vi "Create_Graph_v1.4.vi"() -> ()   [LabVIEW 2018]
uses:
  <vilib>/Native 3D Graph/xcontrol/3DPC_SurfacePlot.xctl
  <vilib>/Native 3D Graph/classes/Base Datatype.lvclass
panel:
  out "3D Graph":refnum<class "Base Datatype.lvclass">[](xcontrol)
  out "Array 2":dbl[][](array[numeric])
  in  "Open":bool
  in  "Загрузка Excel приложения":refnum<k7>
  in  "Excel._Worksheet 2":refnum<k7>
  in  "Array":string[][](array[string])
  in  "Выбор файла":path
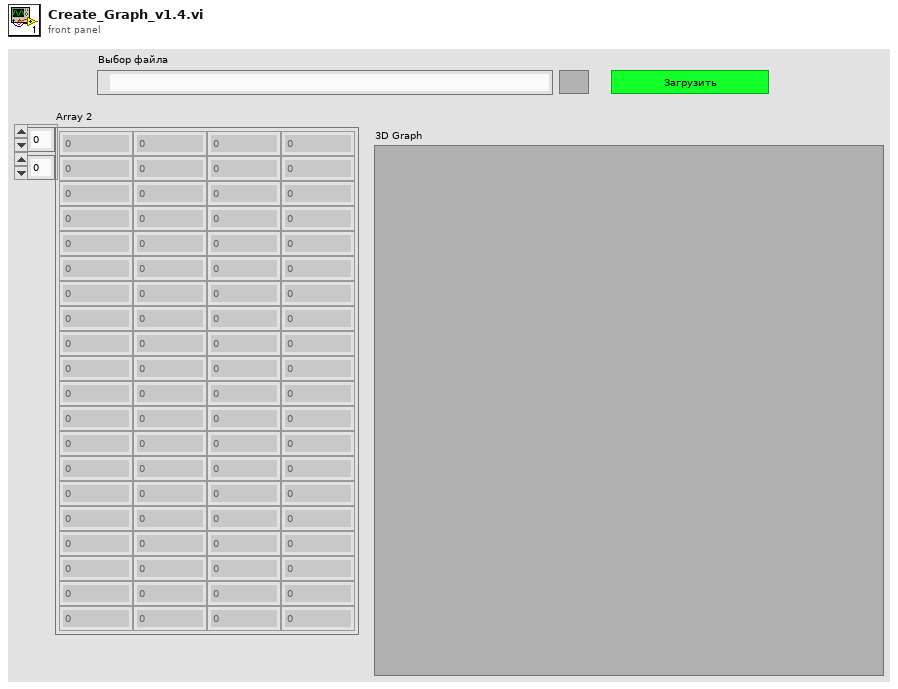
[diagram p1: front panel]
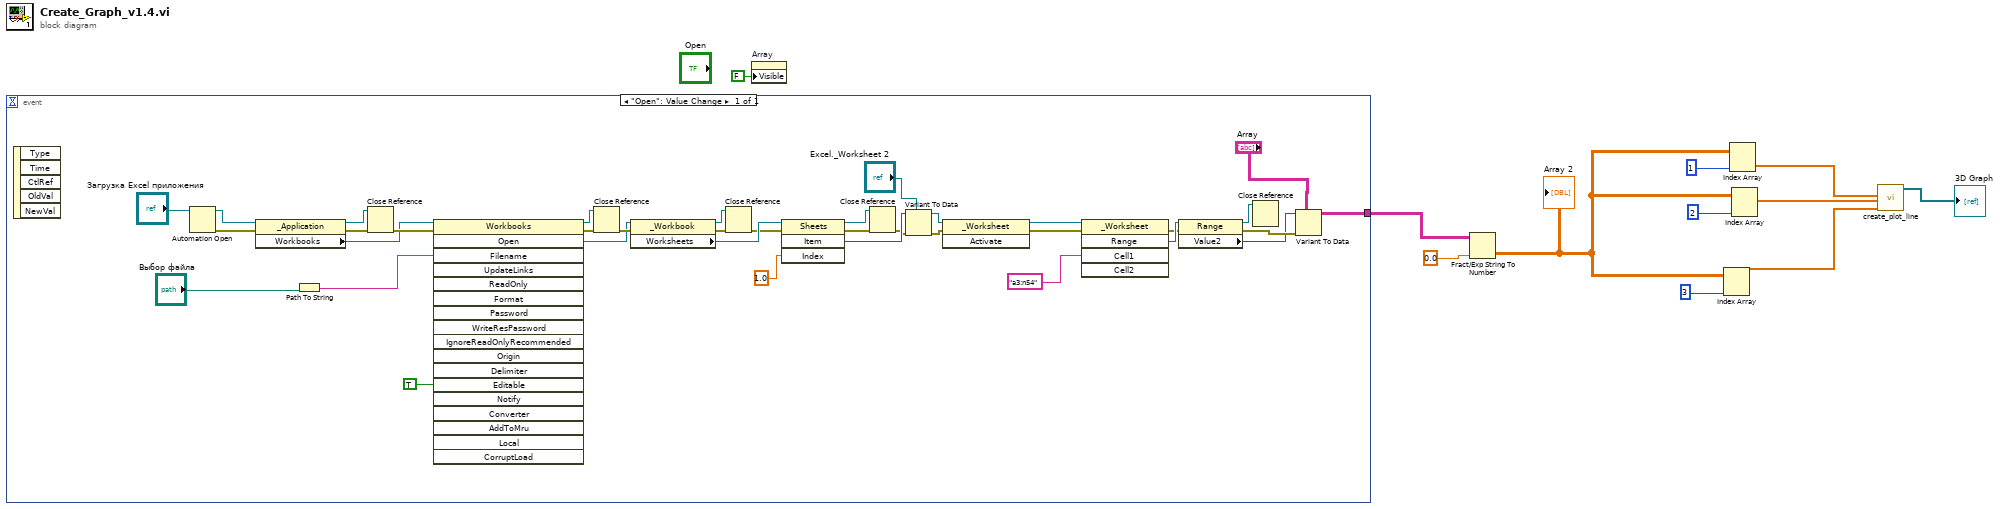
[diagram p0: block diagram]
diagram:
  n1 = event shown="[0] \"Open\": Value Change" {
    selector: _ -> [_]
    dyn-events: _ -> [_]
    timeout: _ -> [_]
    tunnel: [w15] -> w9
    event "Open": Value Change {
      n2 = event-data() -> ()  [unwired: 1 in, 5 out]
      n3 = Automation Open(Automation Refnum="Загрузка Excel приложения") -> (Automation Refnum=w47:refnum<k7>, error out=w35:errorcluster)  [unwired: 3 in]
      n4 = property class="_Application"(reference=w47, error in=w35) -> (reference out=w33:refnum<k7>, error out=w28:errorcluster, "Workbooks"=w18:refnum<k7>)
      n5 = Path To String(path="Выбор файла") -> (string=w16:string)
      n6 = Close Reference(reference=w33, error in (no error)=w28) -> (error out=w27:errorcluster)
      n7 = invoke class="Workbooks" method="Open"(reference=w18, error in=w27, "Filename"=w16, "Editable"=TRUE) -> (reference out=w32:refnum<k7>, error out=w26:errorcluster, "Open"=w17:refnum<k7>)  [unwired: 14 in, 15 out]
      n8 = Close Reference(reference=w32, error in (no error)=w26) -> (error out=w25:errorcluster)
      n9 = property class="_Workbook"(reference=w17, error in=w25) -> (reference out=w31:refnum<k7>, error out=w24:errorcluster, "Worksheets"=w42:refnum<k7>)
      n10 = Close Reference(reference=w31, error in (no error)=w24) -> (error out=w23:errorcluster)
      n11 = invoke class="Sheets" method="Item"(reference=w42, error in=w23, "Index"=1.0) -> (reference out=w30:refnum<k7>, error out=w22:errorcluster, "Item"=w43:variant)  [unwired: 1 in, 1 out]
      n12 = Close Reference(reference=w30, error in (no error)=w22) -> (error out=w21:errorcluster)
      n13 = Variant To Data(error in=w21, type="Excel._Worksheet 2", Variant=w43) -> (data=w45:refnum<k7>, error out=w34:errorcluster)
      n14 = invoke class="_Worksheet" method="Activate"(reference=w45, error in=w34) -> (reference out=w36:refnum<k7>, error out=w20:errorcluster)  [unwired: 1 in, 1 out]
      n15 = invoke class="_Worksheet" method="Range"(reference=w36, error in=w20, "Cell1"="a3:n54") -> (error out=w19:errorcluster, "Range"=w38:refnum<k7>)  [unwired: 2 in, 3 out]
      n16 = property class="Range"(reference=w38, error in=w19) -> (reference out=w29:refnum<k7>, error out=w40:errorcluster, "Value2"=w39:variant)
      n17 = Close Reference(reference=w29) -> ()  [unwired: 1 in, 1 out]
      n18 = Variant To Data(error in=w40, type="Array", Variant=w39) -> (data=w15:string[][])  [unwired: 1 out]
    }
  }
  n19 = property on="Array" class="Arr (strict)"("Visible"=FALSE) -> ()  [unwired: 2 in, 2 out]
  n20 = Fract/Exp String To Number(string=w9, default (0 dbl)=0.0) -> (number=w4:dbl[][])  [unwired: 2 in, 1 out]
  "Array 2" <- w4
  n21 = Index Array(array=w4, index (col)=3) -> (element=w3:dbl[])  [unwired: 1 in]
  n22 = Index Array(array=w4, index (col)=1) -> (element=w1:dbl[])  [unwired: 1 in]
  n23 = Index Array(array=w4, index (col)=2) -> (element=w2:dbl[])  [unwired: 1 in]
  n24 = call <vilib>:"create_plot_line.vi"("z vector"=w3, "y vector"=w2, "x vector"=w1) -> ("plots out"=→"3D Graph":refnum<class "Base Datatype.lvclass">[])  [unwired: 2 in, 6 out]
